vi "Add user inputs to variable array.vi"(8 "error in (no error)":errorcluster, 11 "UserInputs":T1) -> (0 "error out":errorcluster, 3 "UserInputs array":T2)   [LabVIEW 2011]
uses:
  Variable cluster.ctl
  user project design.ctl
panel:
  out "String of available variables":string
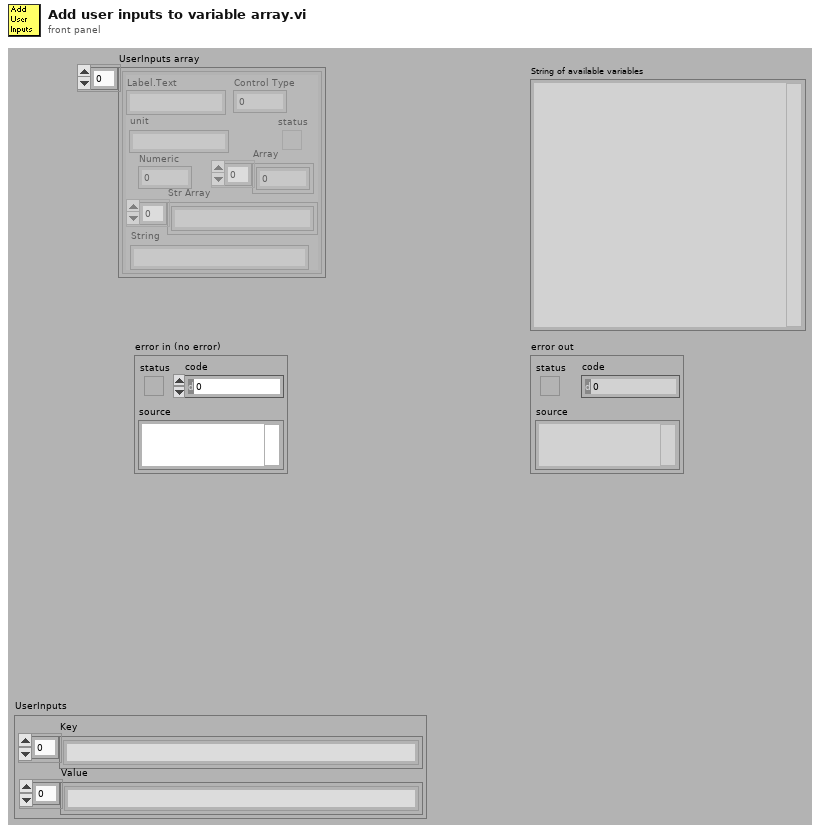
[diagram p1: front panel]
types:
  T1 = typedef "user project design.ctl" = cluster{"Key":string[], "Value":string[]}
  T2 = typedef "Variable cluster.ctl" = cluster{"Label.Text":string, "Control Type":u32, "Numeric":dbl, "Array":dbl[], "status":bool, "Str Array":string[], "String":string, "unit":string}[]
  T3 = cluster{"Label.Text":string, "Caption.Text":string[], "Control Type":u32, "Numeric":dbl, "Array":dbl[], "status":bool, "Outputs":bool[], "Str Array":string[], "String":string}[]
  T4 = cluster{"Label.Text":string, "Control Type":u32, "Numeric":dbl, "Array":dbl[], "status":bool, "Str Array":string[], "String":string, "unit":string}
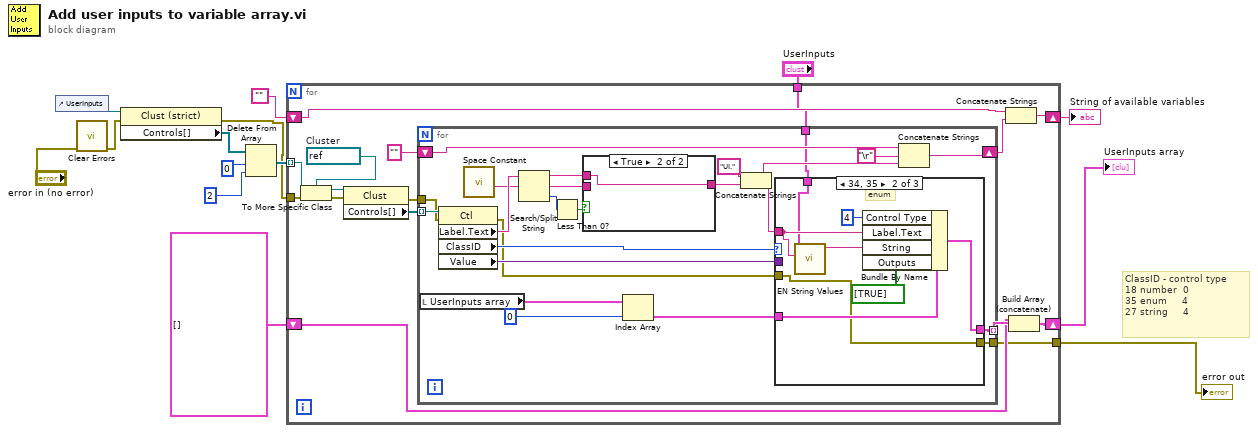
[diagram p0: block diagram]
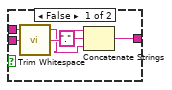
[diagram p2: hidden frame]
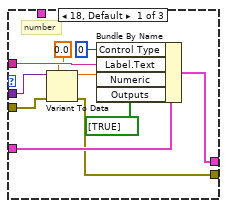
[diagram p3: hidden frame]
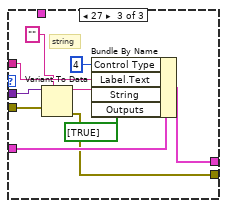
[diagram p4: hidden frame]
diagram:
  # "ClassID - control type\n18 number  0\n35 enum     4\n27 string     4"
  n1 = control-ref of="UserInputs"() -> (w13:refnum<vi>)
  n2 = call <vilib>:"Clear Errors.vi"("error in (no error)"="error in (no error)") -> ("error out"=w1:errorcluster)  [unwired: 6 in]
  n3 = property on="Property Node" class="Clust (strict)"(reference=w13, error in=w1) -> (error out=w4:errorcluster, "Controls[]"=w10:refnum<vi>[])  [unwired: 1 out]
  n4 = Delete From Array(array=w10, length=0 ("index"), index=2) -> (array with subset deleted=w11:refnum<vi>[])  [unwired: 1 out]
  n5 = for {
    tunnel: w11 -> [w29] mode=indexing
    shift-right: [w24] -> w14
    shift-left: T3 [] -> [w23]
    shift-right: [w22] -> w7
    shift-left: "" -> [w21]
    tunnel: w4 -> [w18]
    tunnel: [w16] -> w3
    tunnel: "UserInputs" -> [w15]
    w30 = refnum<vi> refnum  # Cluster
    n6 = To More Specific Class(target class=w30, reference=w29, error in=w18) -> (specific class reference=w27:refnum<vi>, error out=w28:errorcluster)
    n7 = property class="Clust"(reference=w27, error in=w28) -> (error out=w17:errorcluster, "Controls[]"=w26:refnum<vi>[])  [unwired: 1 out]
    n8 = for {
      tunnel: w26 -> [w53] mode=indexing
      tunnel: [w51] -> w25 mode=indexing
      shift-right: [w37] -> w20
      shift-left: "" -> [w38]
      tunnel: w17 -> [w34]
      tunnel: [w32] -> w16
      tunnel: w15 -> [w31]
      n9 = local read "UserInputs array"() -> (w49:T2)
      n10 = property class="Ctl"(reference=w53, error in=w34) -> (error out=w33:errorcluster, "Label.Text"=w45:string, "ClassID"=w52:u32, "Value"=w50:variant)  [unwired: 1 out]
      n11 = call <vilib>:"Space Constant.vi"() -> ("String"=w44:string)
      n12 = Search/Split String(string=w45, search string/char (-)=w44) -> (substring before match=w43:string, match + rest of string=w46:string, offset of match=w41:i32)  [unwired: 1 in]
      n13 = Less Than 0?(x=w41) -> (x < 0?=w40:bool)
      n14 = case shown="True" w40 {
        tunnel: w46 -> [w58 _]
        tunnel: w43 -> [w55 w59]
        tunnel: [w54 w59] -> w42
        frame False {
          n15 = call <vilib>:"Trim Whitespace.vi"("string"=w58) -> ("trimmed string"=w57:string)  [unwired: 1 in]
          n16 = Concatenate Strings(w57, "." ("string"), w55) -> (w54:string)
        }
        frame True {
        }
      }
      n17 = Index Array(array=w49, index=0) -> (element=w47:T4)
      n18 = Concatenate Strings("UI." ("string"), w42) -> (w36:string)
      n19 = case shown="34, 35" w52 {
        tunnel: [w64 w76 w87] -> w51
        tunnel: w36 -> [w68 w73 w86]
        tunnel: w50 -> [w67 _ w85]
        tunnel: w47 -> [w65 w77 w82]
        tunnel: w33 -> [w62 w71 w80]
        tunnel: [w61 w71 w79] -> w32
        tunnel: w31 -> [_ w70 _]
        frame 18, Default {
          # "number"
          n20 = Variant To Data(error in=w62, type=0.0 ("Numeric"), Variant=w67) -> (data=w69:dbl, error out=w61:errorcluster)
          n21 = Bundle By Name(cluster=w65, "Control Type"=u32 0, "Label.Text"=w68, "Numeric"=w69, "Outputs"=bool[] [TRUE]) -> (w64:T4)
        }
        frame 34, 35 {
          # "enum"
          n22 = call "EN String Values.vi"("Label.Text"=w73, "UserInputs"=w70) -> ("String"=w72:string)  [unwired: 9 in]
          n23 = Bundle By Name(cluster=w77, "Control Type"=u32 4, "Label.Text"=w73, "String"=w72, "Outputs"=bool[] [TRUE]) -> (w76:T4)
        }
        frame 27 {
          # "string"
          n24 = Variant To Data(error in=w80, type="" ("String"), Variant=w85) -> (data=w83:string, error out=w79:errorcluster)
          n25 = Bundle By Name(cluster=w82, "Control Type"=u32 4, "Label.Text"=w86, "String"=w83, "Outputs"=bool[] [TRUE]) -> (w87:T4)
        }
      }
      n26 = Concatenate Strings(w38, "\r", w36) -> (w37:string)
    }
    n27 = Concatenate Strings(w21, w20) -> (w22:string)
    n28 = Build Array (concatenate)(w23, w25) -> (w24:T3)
  }
  "UserInputs array" <- w14
  "String of available variables" <- w7
  "error out" <- w3
